vi "Ejecutor_manual.vi"() -> ()   [LabVIEW 2017]
uses:
  GlobalFag.vi
  Global_comSerie.vi
  <vilib>/Instr/_visa.llb/VISA Configure Serial Port (Instr).vi
panel:
  in  "x":u8
  out "sh_reg2":u8
  out "sh_reg":u8
  in  "act_vac":bool
  out "aula":string
  out "estado 3":bool[](array[boolean])
  out "aula_str":string
  out "Edif_":string
  out "estado 2":bool[](array[boolean])
  out "A_fin":u8
  in  "Tab Control":enum32{"Aula", "Edificio"}(tab)
  in  "+                 -":bool
  in  "edo_actual_aula":bool
  in  "stop_aula":bool
  in  "Enviar":bool
  in  "Servicios":bool[](array[boolean])
  in  "Edificio":enum8{"A", "B", "C", "D", "E"}(ring)
  in  "Aula":T1(ring)
  in  "Estado":bool
  out "estado":bool[](array[boolean])
  in  "Hasta":u8=16 min=1 max=16 step=1
  in  "De":u8=1 min=1 max=16 step=1
  in  "rango":bool
  out "Loading":bool
  in  "Enviar 3":bool
  in  "Edificio 2":enum8{"A", "B", "C", "D", "E"}(ring)
  in  "Ser edif":bool[](array[boolean])
  in  "stop_edificio 2":bool
  in  "+_-_edo_actual_edif":bool=TRUE
  in  "+                 -       2":bool
  # "+/- Edo. Actual"
  # "Conf para Edif A, aula 15"
  # "Estado Actual"
  # "Servicio"
  # "Luz"
  # "Luz"
  # "Aire"
  # "Aire"
  # "Proyector"
  # "Proyector"
  # "Agua"
  # "Agua"
  # "Acceso"
  # "Acceso"
  # "+/- Edo Actual"
  # "Servicio"
  # "Aplicar a un rango"
  # "Luz"
  # "Aire"
  # "Proyector"
  # "Agua"
  # "Acceso"
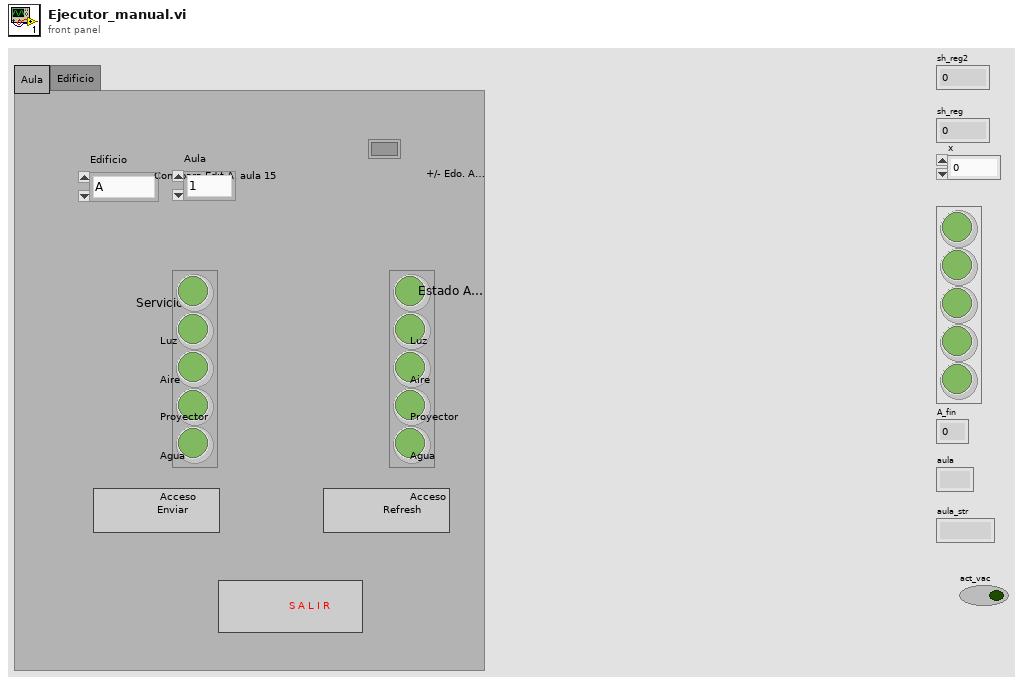
[diagram p1: front panel]
types:
  T1 = enum8{"1", "2", "3", "4", "5", "6", "7", "8", "9", "10", "11", "12", "13", "14", "15", "16"}
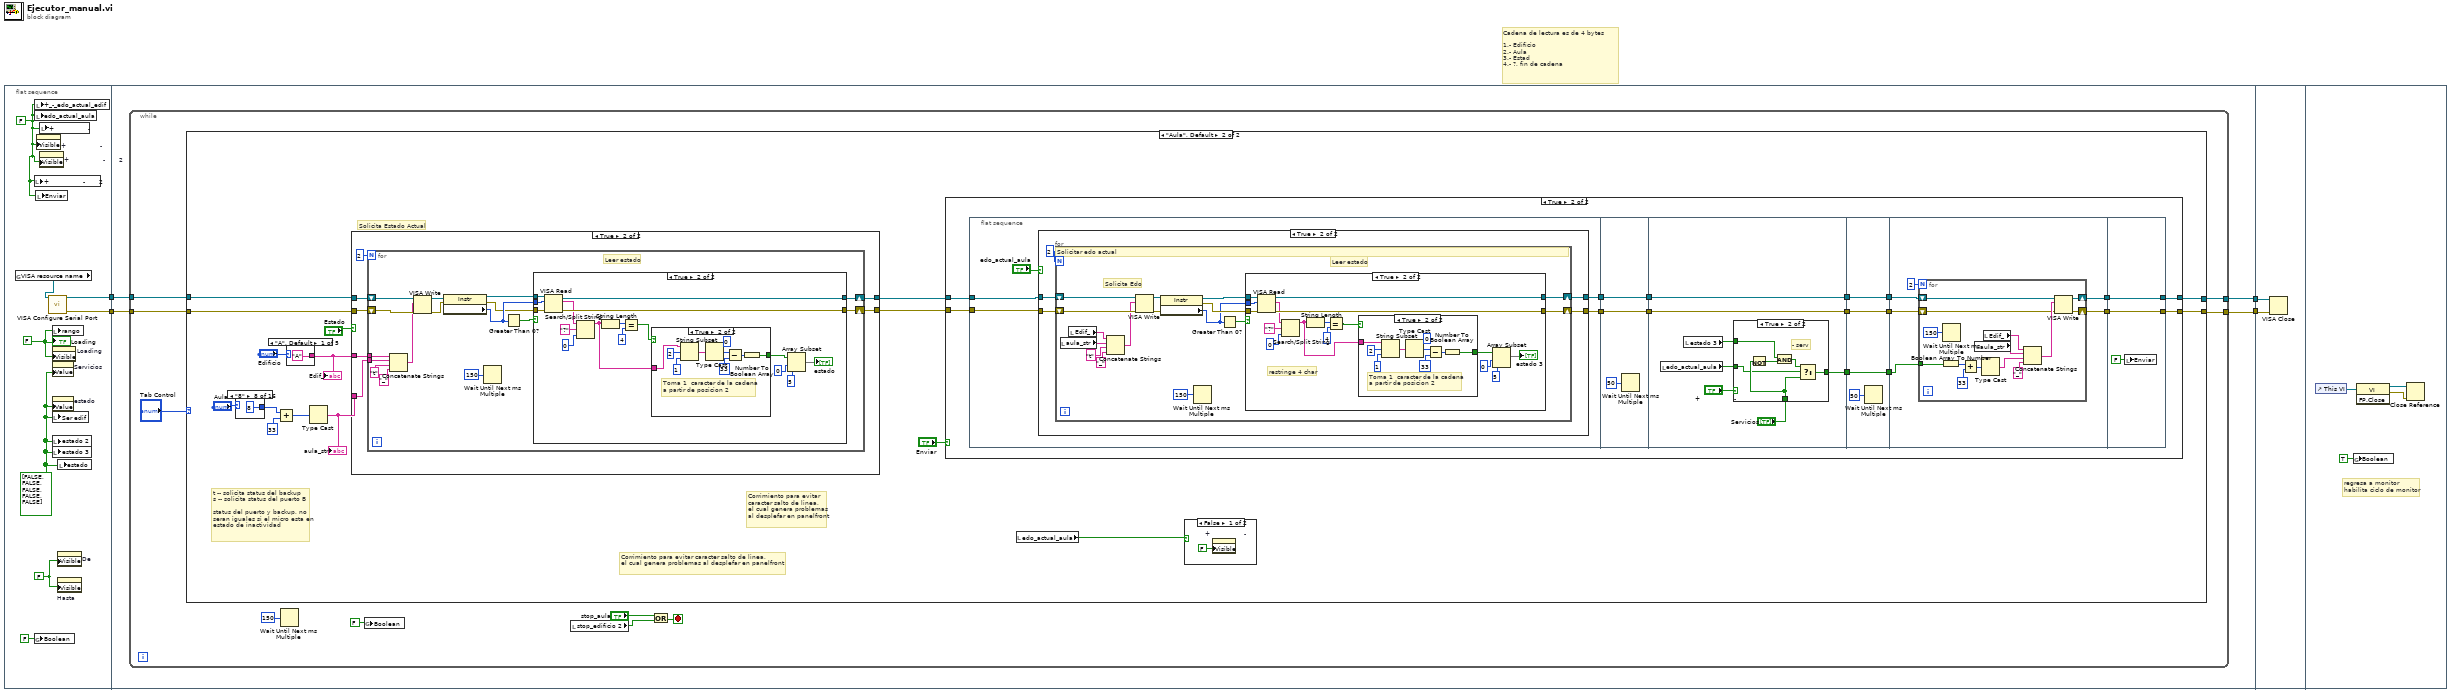
[diagram p0: block diagram]
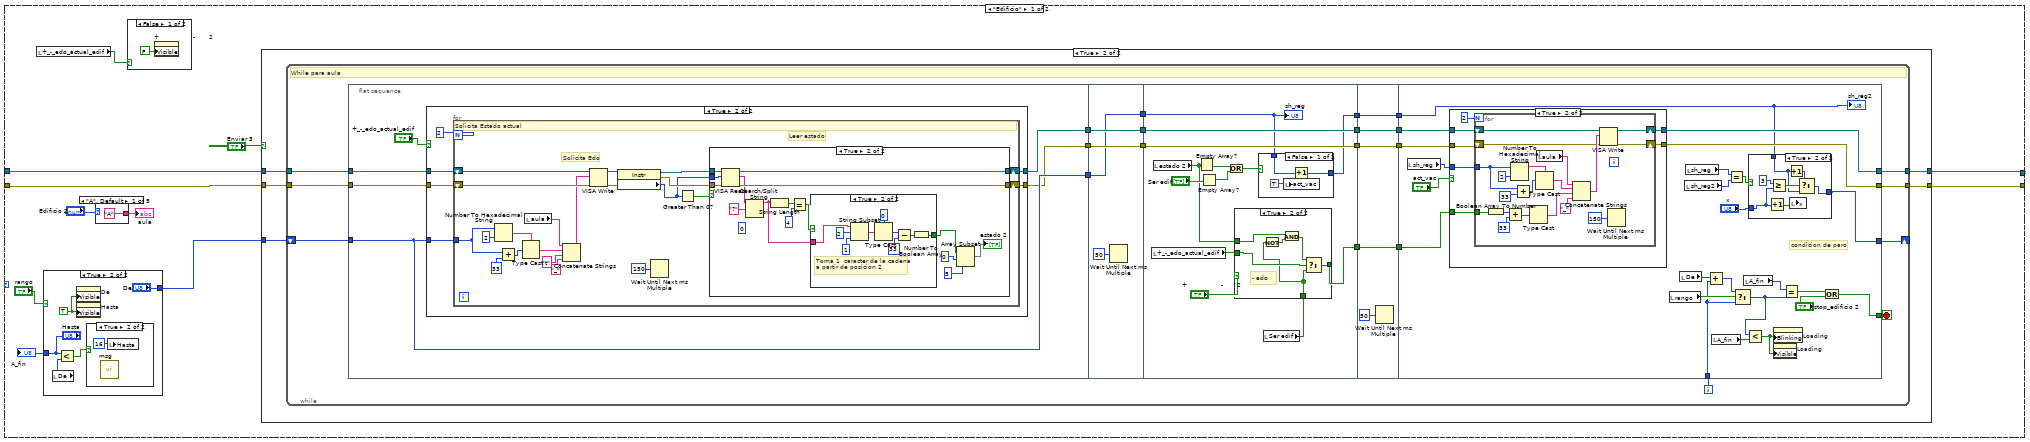
[diagram p2: hidden frame]
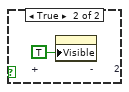
[diagram p3: hidden frame]
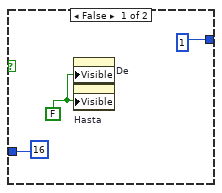
[diagram p4: hidden frame]
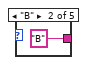
[diagram p6: hidden frame]
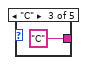
[diagram p7: hidden frame]
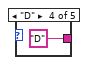
[diagram p8: hidden frame]
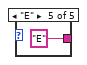
[diagram p9: hidden frame]
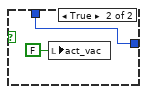
[diagram p14: hidden frame]
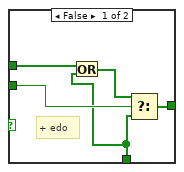
[diagram p15: hidden frame]
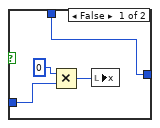
[diagram p16: hidden frame]
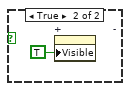
[diagram p18: hidden frame]
diagram:
  # "Cadena de lectura es de 4 bytes\n\n1.- Edificio\n2.- Aula\n3.- Estad\n4.- ?, fin de cadena"
  n1 = flat-sequence {
    tunnel: [w12] -> w4
    tunnel: [w11] -> w3
    tunnel: w4 -> [w16]
    tunnel: w3 -> [w15]
    tunnel: [w14] -> w2
    tunnel: [w13] -> w1
    tunnel: w2 -> [w458]
    tunnel: w1 -> [w457]
    frame #0 {
      w6 = FALSE ("Loading")
      w8 = FALSE
      w9 = FALSE ("Loading")
      w7 = bool[] [FALSE, FALSE, FALSE, FALSE, FALSE] ("Servicios")
      n2 = global read "Global_comSerie.vi" "VISA resource name"() -> (w10:refnum<visa-resource-name>)
      n3 = local write "+                 -       2"(w6) -> ()
      n4 = global write "GlobalFag.vi" "Boolean"(FALSE ("Boolean")) -> ()
      n5 = local write "+_-_edo_actual_edif"(w6) -> ()
      n6 = local write "edo_actual_aula"(w6) -> ()
      n7 = local write "Enviar"(w6) -> ()
      n8 = property on="+                 -" class="Bool (strict)"("Visible"=w6) -> ()  [unwired: 2 in, 2 out]
      n9 = local write "+                 -"(w6) -> ()
      n10 = property on="+                 -       2" class="Bool (strict)"("Visible"=w6) -> ()  [unwired: 2 in, 2 out]
      n11 = call-poly "VISA Configure Serial Port"("VISA resource name"=w10) -> ("VISA resource name out"=w12:refnum<visa-resource-name>, "error out"=w11:errorcluster)  [unwired: 13 in]
      n12 = local write "rango"(w9) -> ()
      n13 = property on="Loading" class="Bool (strict)"("Visible"=w9) -> ()  [unwired: 2 in, 2 out]
      n14 = property on="Servicios" class="Arr (strict)"("Value"=w7) -> ()  [unwired: 2 in, 2 out]
      n15 = property on="estado" class="Arr (strict)"("Value"=w7) -> ()  [unwired: 2 in, 2 out]
      n16 = local write "Ser edif"(w7) -> ()
      n17 = local write "estado 2"(w7) -> ()
      n18 = local write "estado 3"(w7) -> ()
      n19 = property on="De" class="DigNum (strict)"("Visible"=w8) -> ()  [unwired: 2 in, 2 out]
      n20 = property on="Hasta" class="DigNum (strict)"("Visible"=w8) -> ()  [unwired: 2 in, 2 out]
      n21 = local write "estado"(w7) -> ()
      "Loading" <- w9
    }
    frame #1 {
      n22 = while {
        tunnel: w16 -> [w24]
        tunnel: w15 -> [w23]
        tunnel: [w22] -> w14
        tunnel: [w21] -> w13
        stop <- w20 stop-if-true
        n23 = case shown="\"Aula\", Default" "Tab Control" {
          tunnel: w24 -> [w36 w254]
          tunnel: w23 -> [w37 w253]
          tunnel: [w35 w248] -> w22
          tunnel: [w30 w249] -> w21
          frame "Edificio" {
            n24 = local read "+_-_edo_actual_edif"() -> (w27:bool)
            n25 = case shown="True" "rango" {
              tunnel: [u8 1 ("width (-)") "De"] -> w29
              tunnel: [u8 16 "Hasta"] -> w31
              frame False {
                w41 = FALSE
                n26 = property on="De" class="DigNum (strict)"("Visible"=w41) -> ()  [unwired: 2 in, 2 out]
                n27 = property on="Hasta" class="DigNum (strict)"("Visible"=w41) -> ()  [unwired: 2 in, 2 out]
              }
              frame True {
                w47 = TRUE
                n28 = local read "De"() -> (w44:u8)
                n29 = Less?(x="Hasta", y=w44) -> (x < y?=w43:bool)
                n30 = property on="De" class="DigNum (strict)"("Visible"=w47) -> ()  [unwired: 2 in, 2 out]
                n31 = property on="Hasta" class="DigNum (strict)"("Visible"=w47) -> ()  [unwired: 2 in, 2 out]
                n32 = case shown="True" w43 {
                  frame False {
                  }
                  frame True {
                    n33 = call "msg"() -> ()  [unwired: 10 in, 2 out]
                    n34 = local write "Hasta"(u8 16) -> ()
                  }
                }
              }
            }
            "A_fin" <- w31
            n35 = case shown="\"A\", Default" "Edificio 2" {
              tunnel: ["A" "B" "C" "D" "E"] -> w28
              frame "A", Default {
              }
              frame "B" {
              }
              frame "C" {
              }
              frame "D" {
              }
              frame "E" {
              }
            }
            "aula" <- w28
            n36 = case shown="False" w27 {
              frame False {
                n37 = property on="+                 -       2" class="Bool (strict)"("Visible"=FALSE) -> ()  [unwired: 2 in, 2 out]
              }
              frame True {
                n38 = property on="+                 -       2" class="Bool (strict)"("Visible"=TRUE) -> ()  [unwired: 2 in, 2 out]
              }
            }
            n39 = case shown="True" "Enviar 3" {
              tunnel: w37 -> [w54 w60]
              tunnel: w36 -> [w55 w59]
              tunnel: [w54 w58] -> w35
              tunnel: [w55 w57] -> w30
              tunnel: w29 -> [_ w56]
              frame False {
              }
              frame True {
                n40 = while {
                  tunnel: w59 -> [w82]
                  tunnel: w60 -> [w81]
                  tunnel: [w80] -> w57
                  shift-right: [w76] -> _
                  shift-left: w56 -> [w75]
                  tunnel: [w79] -> w58
                  i -> [w77]
                  stop <- w78 stop-if-true
                  # "While para aula"
                  n41 = flat-sequence {
                    tunnel: [w86] -> w74
                    tunnel: w75 -> [w86]
                    tunnel: w81 -> [w87]
                    tunnel: w82 -> [w88]
                    tunnel: [w85] -> w72
                    tunnel: [w84] -> w70
                    tunnel: w74 -> [w144]
                    tunnel: [w144] -> w73
                    tunnel: w72 -> [w147]
                    tunnel: [w147] -> w71
                    tunnel: w70 -> [w146]
                    tunnel: [w146] -> w69
                    tunnel: [w151] -> w68
                    tunnel: w73 -> [w152]
                    tunnel: [w160] -> w66
                    tunnel: [w159] -> w64
                    tunnel: w71 -> [w159]
                    tunnel: [w158] -> w62
                    tunnel: w69 -> [w158]
                    tunnel: w68 -> [w181]
                    tunnel: [w181] -> w67
                    tunnel: w66 -> [w180]
                    tunnel: [w180] -> w65
                    tunnel: w64 -> [w179]
                    tunnel: [w179] -> w63
                    tunnel: w62 -> [w178]
                    tunnel: [w178] -> w61
                    tunnel: [w205] -> w80
                    tunnel: [w204] -> w79
                    tunnel: [w202] -> w78
                    tunnel: w77 -> [w190]
                    tunnel: [w182] -> w76
                    tunnel: w67 -> [w183]
                    tunnel: w65 -> [w193]
                    tunnel: w63 -> [w192]
                    tunnel: w61 -> [w191]
                    frame #0 {
                      n42 = case shown="True" "+_-_edo_actual_edif" {
                        tunnel: [w90 w96] -> w85
                        tunnel: [w89 w95] -> w84
                        tunnel: w88 -> [w90 w94]
                        tunnel: w87 -> [w89 w93]
                        tunnel: w86 -> [_ w91]
                        frame False {
                        }
                        frame True {
                          n43 = for {
                            N: 2 -> [_]
                            tunnel: w91 -> [w99]
                            shift-right: [w115] -> w96
                            shift-left: w94 -> [w113]
                            shift-right: [w114] -> w95
                            shift-left: w93 -> [w112]
                            # "Solicita Edo"
                            # "Leer estado"
                            # "Solicita Estado actual"
                            n44 = Number To Hexadecimal String(1:u8 2 ("width (-)"), 2:w99) -> (0:w101:string)
                            n45 = Add(x=w99, y=u8 33 ("width (-)")) -> (x+y=w103:u8)
                            n46 = Type Cast(type=w101, x=w103) -> (*(type *) &x=w98:string)
                            n47 = local read "aula"() -> (w97:string)
                            n48 = Concatenate Strings(w97, w98, "t" ("string"), "_" ("string")) -> (w111:string)
                            n49 = VISA Write(VISA resource name=w113, write buffer=w111, error in (no error)=w112) -> (VISA resource name out=w116:refnum<visa-resource-name>, error out=w117:errorcluster)  [unwired: 1 out]
                            n50 = property class="Instr"(reference=w116, error in=w117) -> (reference out=w106:refnum<visa-resource-name>, error out=w105:errorcluster, "Serial Settings:Number of Bytes at Serial Port"=w104:u32)
                            n51 = Wait Until Next ms Multiple(millisecond multiple=u32 150) -> ()  [unwired: 1 out]
                            n52 = Greater Than 0?(x=w104) -> (x > 0?=w107:bool)
                            n53 = case shown="True" w107 {
                              tunnel: w106 -> [w118 w134]
                              tunnel: w105 -> [w119 w133]
                              tunnel: [w119 w132] -> w114
                              tunnel: [w118 w131] -> w115
                              tunnel: w104 -> [_ w130]
                              frame False {
                              }
                              frame True {
                                (unwired) u8 0 ("offset (0)")
                                n54 = VISA Read(VISA resource name=w134, byte count=w130, error in (no error)=w133) -> (VISA resource name out=w131:refnum<visa-resource-name>, read buffer=w126:string, error out=w132:errorcluster)  [unwired: 1 out]
                                n55 = Search/Split String(string=w126, search string/char (-)="?") -> (substring before match=w124:string)  [unwired: 1 in, 2 out]
                                n56 = String Length(string=w124) -> (length=w129:i32)
                                n57 = Equal?(x=w129, y=4) -> (x = y?=w125:bool)
                                n58 = case shown="True" w125 {
                                tunnel: [_ w136] -> w123
                                tunnel: w124 -> [_ w135]
                                frame False {
                                }
                                frame True {
                                # "Toma 1  caracter de la cadena\na partir de posicion 2"
                                n59 = String Subset(string=w135, offset (0)=2, length (rest)=1 ("length (rest)")) -> (substring=w140:string)
                                n60 = Type Cast(type=u8 0 ("width (-)"), x=w140) -> (*(type *) &x=w138:u8)
                                n61 = Subtract(x=w138, y=u8 33) -> (x-y=w139:u8)
                                n62 = Number To Boolean Array(number=w139) -> (Boolean array=w136:bool[])
                                }
                                }
                                n63 = Array Subset(array=w123, index=0, length=5) -> (→"estado 2":bool[])
                              }
                            }
                          }
                        }
                      }
                    }
                    frame #1 {
                      n64 = Wait Until Next ms Multiple(millisecond multiple=u32 50) -> ()  [unwired: 1 out]
                    }
                    frame #2 {
                      n65 = local read "+_-_edo_actual_edif"() -> (w157:bool)
                      n66 = local read "estado 2"() -> (w148:bool[])
                      n67 = Empty Array?(array=w148) -> (empty?=w149:bool)
                      n68 = Empty Array?(array="Ser edif") -> (empty?=w153:bool)
                      n69 = Or(x=w149, y=w153) -> (x .or. y?=w154:bool)
                      n70 = case shown="False" w154 {
                        tunnel: w152 -> [w163 w164]
                        tunnel: [w162 w164] -> w151
                        frame False {
                          n71 = local write "act_vac"(TRUE ("Boolean")) -> ()
                          n72 = Increment(x=w163) -> (x+1=w162:u8)
                        }
                        frame True {
                          n73 = local write "act_vac"(FALSE ("Boolean")) -> ()
                        }
                      }
                      n74 = local read "Ser edif"() -> (w150:bool[])
                      n75 = case shown="True" "+                 -       2" {
                        tunnel: [w170 w176] -> w160
                        tunnel: w157 -> [w168 w173]
                        tunnel: w150 -> [w167 w172]
                        tunnel: w148 -> [w166 w171]
                        frame False {
                          # "+ edo"
                          n76 = Or(x=w166, y=w167) -> (x .or. y?=w169:bool[])
                          n77 = Select(t=w169, s=w168, f=w167) -> (s? t:f=w170:bool[])
                        }
                        frame True {
                          # "- edo"
                          n78 = Not(x=w172) -> (.not. x?=w175:bool[])
                          n79 = And(x=w171, y=w175) -> (x .and. y?=w174:bool[])
                          n80 = Select(t=w174, s=w173, f=w172) -> (s? t:f=w176:bool[])
                        }
                      }
                      "sh_reg" <- w152
                    }
                    frame #3 {
                      n81 = Wait Until Next ms Multiple(millisecond multiple=u32 50) -> ()  [unwired: 1 out]
                    }
                    frame #4 {
                      # "condicion de paro"
                      n82 = local read "sh_reg"() -> (w188:u8)
                      n83 = case shown="True" "act_vac" {
                        tunnel: [w218 w225] -> w205
                        tunnel: [w217 w224] -> w204
                        tunnel: w188 -> [_ w222]
                        tunnel: w193 -> [_ w221]
                        tunnel: w192 -> [w218 w220]
                        tunnel: w191 -> [w217 w219]
                        frame False {
                        }
                        frame True {
                          n84 = for {
                            N: 2 -> [_]
                            tunnel: w221 -> [w229]
                            tunnel: w222 -> [w227]
                            shift-right: [w237] -> w225
                            shift-left: w220 -> [w239]
                            shift-right: [w234] -> w224
                            shift-left: w219 -> [w238]
                            n85 = Boolean Array To Number(Boolean array=w229) -> (number=w233:u8)
                            n86 = Add(x=w233, y=u8 33) -> (x+y=w232:u8)
                            n87 = Number To Hexadecimal String(1:u8 2 ("width (-)"), 2:w227) -> (0:w242:string)
                            n88 = Add(x=w227, y=u8 33 ("width (-)")) -> (x+y=w235:u8)
                            n89 = Type Cast(x=w232) -> (*(type *) &x=w230:string)  [unwired: 1 in]
                            n90 = Type Cast(type=w242, x=w235) -> (*(type *) &x=w244:string)
                            n91 = local read "aula"() -> (w228:string)
                            n92 = Concatenate Strings(w228, w244, w230, "_" ("string")) -> (w240:string)
                            n93 = VISA Write(VISA resource name=w239, write buffer=w240, error in (no error)=w238) -> (VISA resource name out=w237:refnum<visa-resource-name>, error out=w234:errorcluster)  [unwired: 1 out]
                            n94 = Wait Until Next ms Multiple(millisecond multiple=u32 150) -> ()  [unwired: 1 out]
                          }
                        }
                      }
                      n95 = local read "rango"() -> (w197:bool)
                      n96 = local read "De"() -> (w195:u8)
                      n97 = local read "sh_reg2"() -> (w186:u8)
                      n98 = local read "sh_reg"() -> (w187:u8)
                      n99 = Add(x=w195, y=w190) -> (x+y=w196:i32)
                      n100 = local read "A_fin"() -> (w198:u8)
                      n101 = Equal?(x=w187, y=w186) -> (x = y?=w185:bool)
                      n102 = Select(t=w196, s=w197, f=w190) -> (s? t:f=w194:i32)
                      n103 = local read "A_fin"() -> (w199:u8)
                      n104 = Less?(x=w194, y=w198) -> (x < y?=w200:bool)
                      n105 = case shown="True" w185 {
                        tunnel: "x" -> [w209 w215]
                        tunnel: w183 -> [w206 w211]
                        tunnel: [w206 w210] -> w182
                        frame False {
                          n106 = Multiply(x=u8 0, y=w209) -> (x*y=w207:u8)
                          n107 = local write "x"(w207) -> ()
                        }
                        frame True {
                          n108 = Increment(x=w215) -> (x+1=w216:u8)
                          n109 = Greater Or Equal?(x=u8 3, y=w215) -> (x >= y?=w213:bool)
                          n110 = Increment(x=w211) -> (x+1=w212:u8)
                          n111 = local write "x"(w216) -> ()
                          n112 = Select(t=w212, s=w213, f=w211) -> (s? t:f=w210:u8)
                        }
                      }
                      n113 = property on="Loading" class="Bool (strict)"("Blinking"=w200) -> ()  [unwired: 2 in, 2 out]
                      n114 = property on="Loading" class="Bool (strict)"("Visible"=w200) -> ()  [unwired: 2 in, 2 out]
                      n115 = Equal?(x=w199, y=w194) -> (x = y?=w203:bool)
                      n116 = Compound Arithmetic op=OR(w203, "stop_edificio 2") -> (w202:bool)
                      "sh_reg2" <- w183
                    }
                  }
                }
              }
            }
          }
          frame "Aula", Default {
            # "Corrimiento para evitar\ncaracter salto de linea,\nel cual genera problemas\nal desplefar en panelfront"
            # "t -- solicita status del backup\ns -- solicita status del puerto B\n\nstatus del puerto y backup, no \nseran iguales si el micro esta en\nestado de inactividad"
            # "Solicita Estado Actual"
            # "Corrimiento para evitar caracter salto de linea,\nel cual genera problemas al desplefar en panelfront"
            n117 = case shown="\"8\"" "Aula" {
              tunnel: [u8 1 u8 2 u8 3 u8 4 u8 5 u8 6 u8 7 u8 8 u8 9 u8 10 u8 11 u8 12 u8 13 u8 14 u8 15 u8 16] -> w259
              frame "1", Default {
              }
              frame "2" {
              }
              frame "3" {
              }
              frame "4" {
              }
              frame "5" {
              }
              frame "6" {
              }
              frame "7" {
              }
              frame "8" {
              }
              frame "9" {
              }
              frame "10" {
              }
              frame "11" {
              }
              frame "12" {
              }
              frame "13" {
              }
              frame "14" {
              }
              frame "15" {
              }
              frame "16" {
              }
            }
            n118 = Add(x=w259, y=u8 33) -> (x+y=w255:u8)
            n119 = case shown="\"A\", Default" "Edificio" {
              tunnel: ["A" "B" "C" "D" "E"] -> w252
              frame "A", Default {
              }
              frame "B" {
              }
              frame "C" {
              }
              frame "D" {
              }
              frame "E" {
              }
            }
            "Edif_" <- w252
            n120 = Type Cast(x=w255) -> (*(type *) &x=w251:string)  [unwired: 1 in]
            "aula_str" <- w251
            n121 = case shown="True" "Estado" {
              tunnel: w254 -> [w406 w413]
              tunnel: w253 -> [w405 w412]
              tunnel: w252 -> [_ w411]
              tunnel: w251 -> [_ w410]
              tunnel: [w406 w409] -> w246
              tunnel: [w405 w408] -> w245
              frame False {
              }
              frame True {
                n122 = for {
                  N: 2 -> [_]
                  tunnel: w411 -> [w425]
                  tunnel: w410 -> [w424]
                  shift-right: [w416] -> w409
                  shift-left: w413 -> [w429]
                  shift-right: [w415] -> w408
                  shift-left: w412 -> [w428]
                  # "Leer estado"
                  n123 = Concatenate Strings(w425, w424, "t" ("string"), "_" ("string")) -> (w423:string)
                  n124 = VISA Write(VISA resource name=w429, write buffer=w423, error in (no error)=w428) -> (VISA resource name out=w418:refnum<visa-resource-name>, error out=w417:errorcluster)  [unwired: 1 out]
                  n125 = property class="Instr"(reference=w418, error in=w417) -> (reference out=w419:refnum<visa-resource-name>, error out=w420:errorcluster, "Serial Settings:Number of Bytes at Serial Port"=w421:u32)
                  n126 = Wait Until Next ms Multiple(millisecond multiple=u32 150) -> ()  [unwired: 1 out]
                  n127 = Greater Than 0?(x=w421) -> (x > 0?=w422:bool)
                  n128 = case shown="True" w422 {
                    tunnel: w419 -> [w430 w447]
                    tunnel: w420 -> [w431 w446]
                    tunnel: [w431 w445] -> w415
                    tunnel: [w430 w444] -> w416
                    tunnel: w421 -> [_ w443]
                    frame False {
                    }
                    frame True {
                      n129 = VISA Read(VISA resource name=w447, byte count=w443, error in (no error)=w446) -> (VISA resource name out=w444:refnum<visa-resource-name>, read buffer=w439:string, error out=w445:errorcluster)  [unwired: 1 out]
                      n130 = Search/Split String(string=w439, search string/char (-)="?", offset (0)=u8 0) -> (substring before match=w436:string)  [unwired: 2 out]
                      n131 = String Length(string=w436) -> (length=w442:i32)
                      n132 = Equal?(x=w442, y=4) -> (x = y?=w437:bool)
                      n133 = case shown="True" w437 {
                        tunnel: w436 -> [_ w449]
                        tunnel: [_ w448] -> w434
                        frame False {
                        }
                        frame True {
                          # "Toma 1  caracter de la cadena\na partir de posicion 2"
                          n134 = String Subset(string=w449, offset (0)=2, length (rest)=1 ("length (rest)")) -> (substring=w453:string)
                          n135 = Type Cast(type=u8 0 ("width (-)"), x=w453) -> (*(type *) &x=w451:u8)
                          n136 = Subtract(x=w451, y=u8 33) -> (x-y=w452:u8)
                          n137 = Number To Boolean Array(number=w452) -> (Boolean array=w448:bool[])
                        }
                      }
                      n138 = Array Subset(array=w434, index=0, length=5) -> (→"estado":bool[])
                    }
                  }
                }
              }
            }
            n139 = case shown="True" "Enviar" {
              tunnel: w246 -> [w263 w280]
              tunnel: w245 -> [w264 w279]
              tunnel: [w263 w278] -> w249
              tunnel: [w264 w277] -> w248
              frame False {
              }
              frame True {
                n140 = flat-sequence {
                  tunnel: [w285] -> w276
                  tunnel: [w284] -> w274
                  tunnel: w280 -> [w283]
                  tunnel: w279 -> [w282]
                  tunnel: w276 -> [w338]
                  tunnel: [w338] -> w275
                  tunnel: w274 -> [w337]
                  tunnel: [w337] -> w273
                  tunnel: w275 -> [w345]
                  tunnel: [w345] -> w270
                  tunnel: w273 -> [w344]
                  tunnel: [w344] -> w268
                  tunnel: [w342] -> w266
                  tunnel: w270 -> [w360]
                  tunnel: [w360] -> w269
                  tunnel: w268 -> [w359]
                  tunnel: [w359] -> w267
                  tunnel: w266 -> [w358]
                  tunnel: [w358] -> w265
                  tunnel: w269 -> [w366]
                  tunnel: w267 -> [w365]
                  tunnel: w265 -> [w361]
                  tunnel: [w364] -> w272
                  tunnel: [w363] -> w271
                  tunnel: [w382] -> w277
                  tunnel: [w383] -> w278
                  tunnel: w272 -> [w383]
                  tunnel: w271 -> [w382]
                  frame #0 {
                    n141 = case shown="True" "edo_actual_aula" {
                      tunnel: [w287 w292] -> w284
                      tunnel: [w286 w291] -> w285
                      tunnel: w283 -> [w287 w290]
                      tunnel: w282 -> [w286 w289]
                      frame False {
                      }
                      frame True {
                        n142 = for {
                          N: 2 -> [_]
                          shift-right: [w306] -> w292
                          shift-left: w290 -> [w304]
                          shift-right: [w305] -> w291
                          shift-left: w289 -> [w303]
                          # "Solicita Edo"
                          # "Leer estado"
                          # "Solicitar edo actual"
                          n143 = local read "aula_str"() -> (w294:string)
                          n144 = local read "Edif_"() -> (w293:string)
                          n145 = Concatenate Strings(w293, w294, "t" ("string"), "_" ("string")) -> (w302:string)
                          n146 = VISA Write(VISA resource name=w304, write buffer=w302, error in (no error)=w303) -> (VISA resource name out=w307:refnum<visa-resource-name>, error out=w308:errorcluster)  [unwired: 1 out]
                          n147 = property class="Instr"(reference=w307, error in=w308) -> (reference out=w297:refnum<visa-resource-name>, error out=w296:errorcluster, "Serial Settings:Number of Bytes at Serial Port"=w295:u32)
                          n148 = Wait Until Next ms Multiple(millisecond multiple=u32 150) -> ()  [unwired: 1 out]
                          n149 = Greater Than 0?(x=w295) -> (x > 0?=w298:bool)
                          n150 = case shown="True" w298 {
                            tunnel: w297 -> [w309 w326]
                            tunnel: w296 -> [w310 w325]
                            tunnel: [w310 w324] -> w305
                            tunnel: [w309 w323] -> w306
                            tunnel: w295 -> [_ w322]
                            frame False {
                            }
                            frame True {
                              # "restringe 4 char"
                              n151 = VISA Read(VISA resource name=w326, byte count=w322, error in (no error)=w325) -> (VISA resource name out=w323:refnum<visa-resource-name>, read buffer=w318:string, error out=w324:errorcluster)  [unwired: 1 out]
                              n152 = Search/Split String(string=w318, search string/char (-)="?", offset (0)=u8 0) -> (substring before match=w316:string)  [unwired: 2 out]
                              n153 = String Length(string=w316) -> (length=w319:i32)
                              n154 = Equal?(x=w319, y=4) -> (x = y?=w317:bool)
                              n155 = case shown="True" w317 {
                                tunnel: [_ w328] -> w314
                                tunnel: w316 -> [_ w327]
                                frame False {
                                }
                                frame True {
                                # "Toma 1  caracter de la cadena\na partir de posicion 2"
                                n156 = String Subset(string=w327, offset (0)=2, length (rest)=1 ("length (rest)")) -> (substring=w332:string)
                                n157 = Type Cast(type=u8 0 ("width (-)"), x=w332) -> (*(type *) &x=w330:u8)
                                n158 = Subtract(x=w330, y=u8 33) -> (x-y=w331:u8)
                                n159 = Number To Boolean Array(number=w331) -> (Boolean array=w328:bool[])
                                }
                              }
                              n160 = Array Subset(array=w314, index=0, length=5) -> (→"estado 3":bool[])
                            }
                          }
                        }
                      }
                    }
                  }
                  frame #1 {
                    n161 = Wait Until Next ms Multiple(millisecond multiple=u32 50) -> ()  [unwired: 1 out]
                  }
                  frame #2 {
                    n162 = local read "edo_actual_aula"() -> (w339:bool)
                    n163 = local read "estado 3"() -> (w340:bool[])
                    n164 = case shown="True" "+                 -" {
                      tunnel: [w350 w354] -> w342
                      tunnel: "Servicios" -> [w346 w353]
                      tunnel: w340 -> [w348 w352]
                      tunnel: w339 -> [w347 w351]
                      frame False {
                        # "+ serv"
                        n165 = Or(x=w348, y=w346) -> (x .or. y?=w349:bool[])
                        n166 = Select(t=w349, s=w347, f=w346) -> (s? t:f=w350:bool[])
                      }
                      frame True {
                        # "- serv"
                        n167 = Not(x=w353) -> (.not. x?=w356:bool[])
                        n168 = And(x=w352, y=w356) -> (x .and. y?=w355:bool[])
                        n169 = Select(t=w355, s=w351, f=w353) -> (s? t:f=w354:bool[])
                      }
                    }
                  }
                  frame #3 {
                    n170 = Wait Until Next ms Multiple(millisecond multiple=u32 50) -> ()  [unwired: 1 out]
                  }
                  frame #4 {
                    n171 = for {
                      N: 2 -> [_]
                      shift-right: [w369] -> w363
                      shift-left: w366 -> [w376]
                      shift-right: [w370] -> w364
                      shift-left: w365 -> [w375]
                      tunnel: w361 -> [w368]
                      n172 = Boolean Array To Number(Boolean array=w368) -> (number=w373:u8)
                      n173 = Wait Until Next ms Multiple(millisecond multiple=u32 150) -> ()  [unwired: 1 out]
                      n174 = Add(x=w373, y=u8 33) -> (x+y=w374:u8)
                      n175 = local read "aula_str"() -> (w379:string)
                      n176 = Type Cast(x=w374) -> (*(type *) &x=w371:string)  [unwired: 1 in]
                      n177 = local read "Edif_"() -> (w380:string)
                      n178 = Concatenate Strings(w380, w379, w371, "_" ("string")) -> (w378:string)
                      n179 = VISA Write(VISA resource name=w375, write buffer=w378, error in (no error)=w376) -> (VISA resource name out=w370:refnum<visa-resource-name>, error out=w369:errorcluster)  [unwired: 1 out]
                    }
                  }
                  frame #5 {
                    n180 = local write "Enviar"(FALSE ("Enviar")) -> ()
                  }
                }
              }
            }
            n181 = local read "edo_actual_aula"() -> (w247:bool)
            n182 = case shown="False" w247 {
              frame False {
                n183 = property on="+                 -" class="Bool (strict)"("Visible"=FALSE) -> ()  [unwired: 2 in, 2 out]
              }
              frame True {
                n184 = property on="+                 -" class="Bool (strict)"("Visible"=TRUE) -> ()  [unwired: 2 in, 2 out]
              }
            }
          }
        }
        n185 = Wait Until Next ms Multiple(millisecond multiple=u32 150) -> ()  [unwired: 1 out]
        n186 = global write "GlobalFag.vi" "Boolean"(FALSE ("Boolean")) -> ()
        n187 = local read "stop_edificio 2"() -> (w17:bool)
        n188 = Compound Arithmetic op=OR("stop_aula", w17) -> (w20:bool)
      }
    }
    frame #2 {
      n189 = VISA Close(VISA resource name=w457, error in (no error)=w458) -> ()  [unwired: 1 out]
    }
    frame #3 {
      # "regresa a monitor\nhabilita ciclo de monitor"
      n190 = control-ref of="This VI"() -> (w461:refnum<vi>)
      n191 = global write "GlobalFag.vi" "Boolean"(TRUE ("Boolean")) -> ()
      n192 = invoke class="VI" method="FP.Close"(reference=w461) -> (reference out=w459:refnum<vi>, error out=w460:errorcluster)  [unwired: 2 in, 1 out]
      n193 = Close Reference(reference=w459, error in (no error)=w460) -> ()  [unwired: 1 out]
    }
  }
